vi "test Import with Parameters Files Missing Something.vi"(8 "error in":errorcluster, 11 "TestCase in":refnum<class "1553 Parameters Import.lvclass">) -> (0 "error out":errorcluster, 3 "TestCase out":refnum<class "1553 Parameters Import.lvclass">)   [LabVIEW 2020, in "1553 Parameters Import.lvclass"]
uses:
  1553 Parameters Import.lvclass
  <vilib>/addons/_JKI Toolkits/VI Tester/TestCase.llb/TestCase.lvclass
  Import/MIL-STD 1553 Import.lvlib
  C:/Program Files (x86)/National Instruments/LabVIEW 2020/vi.lib/addons/_JKI Toolkits/VI Tester/TestCase.llb/TestCase.lvclass
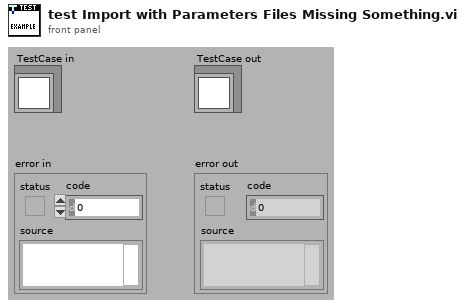
[diagram p1: front panel]
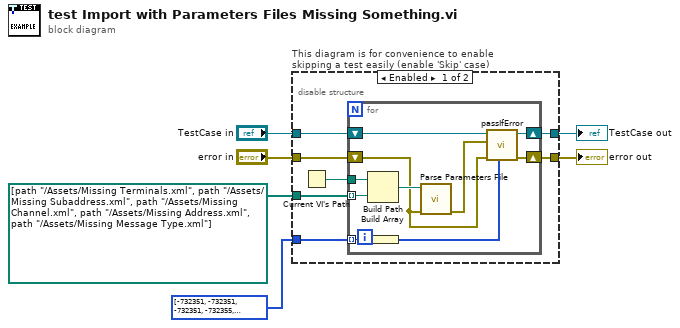
[diagram p0: block diagram]
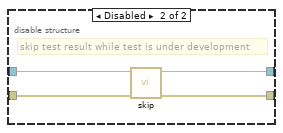
[diagram p2: hidden frame]
diagram:
  n1 = disable-structure "This diagram is for convenience to enable skipping a test easily (enable 'Skip' case)" shown="Enabled" {
    disable-tunnel: "TestCase in" -> [w12 w27]
    disable-tunnel: [w11 w25] -> w3
    disable-tunnel: [w8 w26] -> w5
    disable-tunnel: "error in" -> [w10 w24]
    disable-tunnel: path[] [path "../Assets/Missing Terminals.xml", path "../Assets/Missing Subaddress.xml", path "../Assets/Missing Channel.xml", path "../Assets/Missing Address.xml", path "../Assets/Missing Message Type.xml"] -> [w13 _]
    disable-tunnel: i32[] [-732351, -732351, -732351, -732355, -732351] ("codes") -> [w7 _]
    frame Enabled {
      n2 = Current VI's Path() -> (path=w9:path)
      n3 = for {
        tunnel: w13 -> [w22] mode=indexing
        shift-right: [w19] -> w11
        shift-left: w12 -> [w20]
        shift-right: [w18] -> w8
        shift-left: w10 -> [w17]
        tunnel: w9 -> [w21]
        tunnel: w7 -> [w15] mode=indexing
        n4 = Build Path(base path=w21, name or relative path=w22) -> (appended path=w23:path)
        n5 = Build Array(w15) -> (w14:i32[])
        n6 = call "Parse Parameters File.vi"("error in"=w17, "path to XML document"=w23) -> ("error out"=w16:errorcluster)  [unwired: 7 in, 2 out]
        n7 = call-dynamic "passIfError.vi"("passing error codes (default = any error code)"=w14, "error in (no error)"=w17, "error"=w16, "TestCase in"=w20) -> ("error out"=w18:errorcluster, "TestCase out"=w19:refnum<class "1553 Parameters Import.lvclass">)  [unwired: 6 in]
      }
    }
    frame Disabled {
      # "skip test result while test is under development"
      n8 = call <vilib>:"skip.vi"("error in (no error)"=w24, "TestCase in"=w27) -> ("error out"=w26:errorcluster, "TestCase out"=w25:refnum<class "1553 Parameters Import.lvclass">)  [unwired: 8 in]
    }
  }
  "error out" <- w5
  "TestCase out" <- w3
